vi "Find Specific USB Com Port.vi"(4 "Error In":errorcluster, 7 "Identifiers (regular expressions)":T2={"Vendor ID"="VID_0403", "Product ID"="PID_6001", "S/N"="FTXOVPUUA"}) -> (0 "Error Out":errorcluster, 2 "Device Info":T1={"Service"="FTSER2K", "Manufacturer"="FTDI", "PNPDeviceID"="FTDIBUS\\VID_0403+PID_6001+FTTR2S8CA\\0000"}, 3 "Com Port":refnum<visa-resource-name>)   [LabVIEW 2016]
uses:
  <vilib>/Utility/error.llb/Error Cluster From Error Code.vi
  <vilib>/ErrorRing/Error Ring.xnode
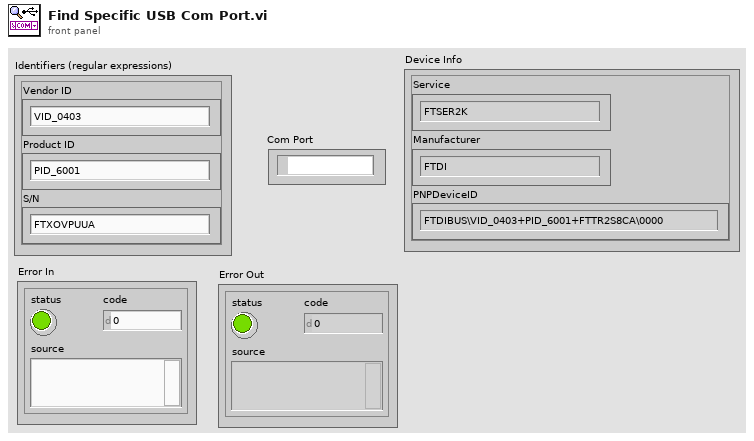
[diagram p1: front panel]
types:
  T1 = cluster{"Service":string, "Manufacturer":string, "PNPDeviceID":string}
  T2 = cluster{"Vendor ID":string, "Product ID":string, "S/N":string}
  T3 = cluster{"Service":string, "Manufacturer":string, "Device":string, "Vendor ID":string, "Product ID":string, "S/N":string, "Instance":string}
  T4 = cluster{"Service":string, "Manufacturer":string, "PNPDeviceID":string}[]
  T5 = cluster{"Name":string, "Caption":string, "Description":string}[]
  T6 = cluster{"Name":string, "Caption":string, "Description":string}
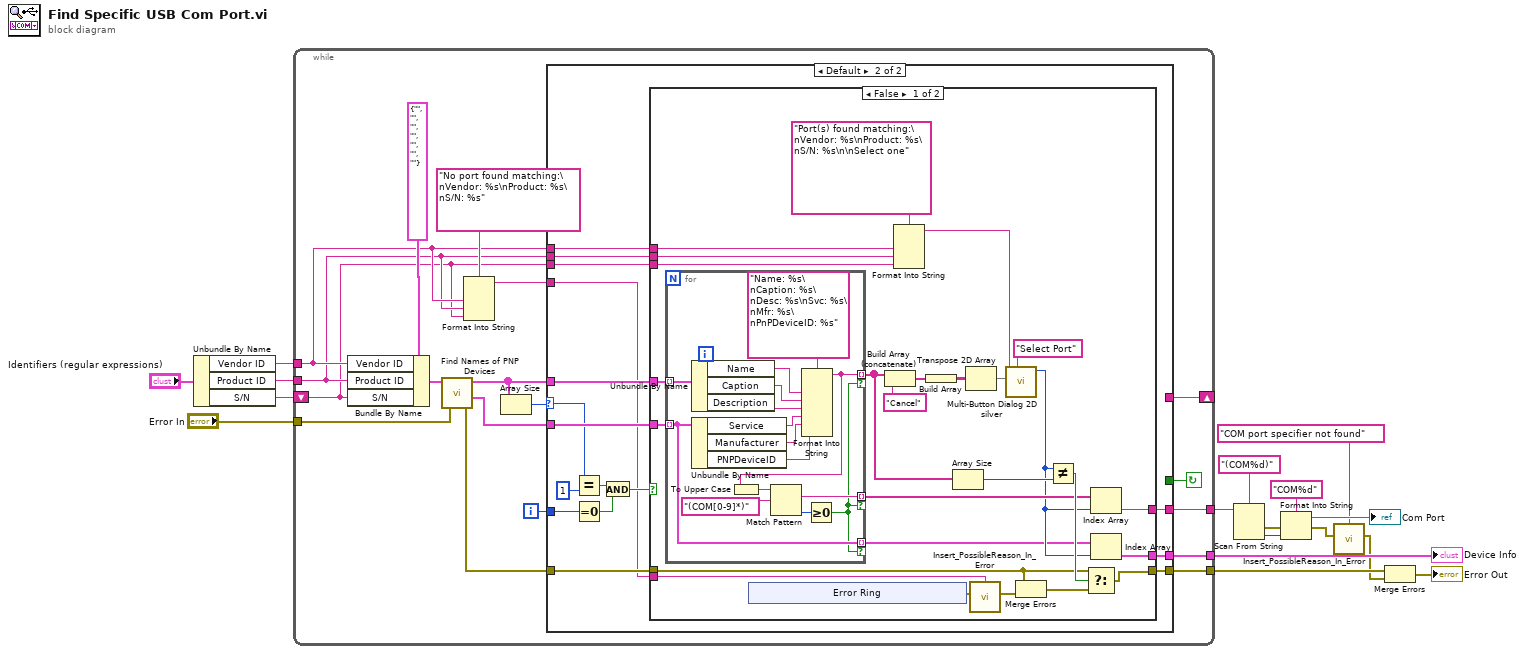
[diagram p0: block diagram]
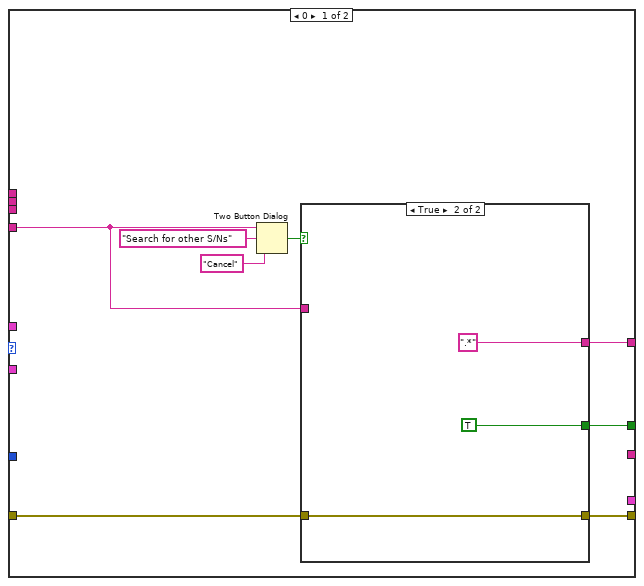
[diagram p2: hidden frame]
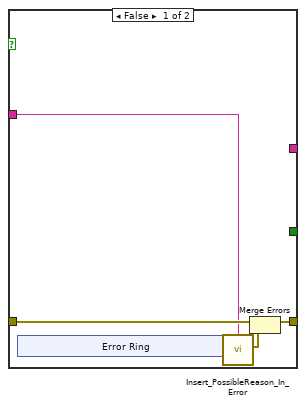
[diagram p3: hidden frame]
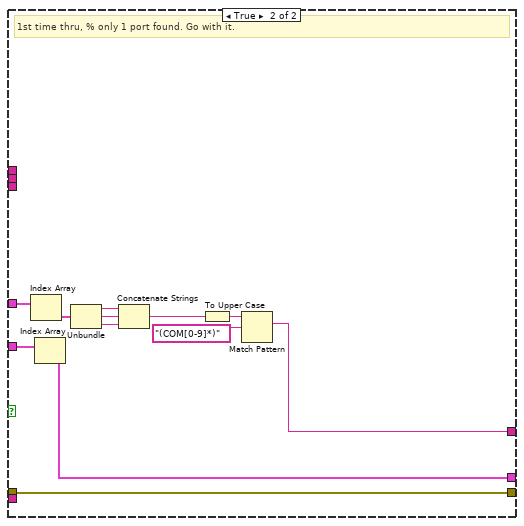
[diagram p4: hidden frame]
diagram:
  n1 = Unbundle By Name("Identifiers (regular expressions)") -> ("Vendor ID"=w15:string, "Product ID"=w14:string, "S/N"=w13:string)
  n2 = while {
    tunnel: "Error In" -> [w26]
    tunnel: w15 -> [w22]
    tunnel: w14 -> [w21]
    shift-right: [w31] -> _
    shift-left: w13 -> [w20]
    tunnel: [w29] -> w12
    tunnel: [w27] -> w11
    tunnel: [w18] -> w2
    i -> [w28]
    stop <- w30 continue-if-true
    n3 = Bundle By Name(cluster=T3 {"Service"="", "Manufacturer"="", "Device"="", "Vendor ID"="", "Product ID"="", "S/N"="", "Instance"=""} ("Identifiers (regular expressions)"), "Vendor ID"=w22, "Product ID"=w21, "S/N"=w20) -> (w34:T3)
    n4 = call "Find Names of PNP Devices.vi"("Error In"=w26, "Identifiers (regular expressions. Use blank to ignore)"=w34) -> ("Error Out"=w25:errorcluster, "Matching Items"=w24:T4, "Names"=w33:T5)  [unwired: 3 in]
    n5 = Format Into String(format string="No port found matching:\nVendor: %s\nProduct: %s\nS/N: %s", w22, w21, w20) -> (resulting string=w19:string)  [unwired: 2 in, 1 out]
    n6 = Array Size(array=w33) -> (size(s)=w32:i32)
    n7 = case shown="Default" w32 {
      selector: w32 -> [_ w65]
      tunnel: w33 -> [_ w68]
      tunnel: w22 -> [_ w71]
      tunnel: w21 -> [_ w70]
      tunnel: w20 -> [_ w69]
      tunnel: w24 -> [_ w67]
      tunnel: [w40 _] -> w31
      tunnel: [w39 _] -> w30
      tunnel: w25 -> [w38 w59]
      tunnel: [w37 w58] -> w29
      tunnel: w28 -> [_ w63]
      tunnel: [_ w60] -> w27
      tunnel: w19 -> [w36 w57]
      tunnel: [_ w56] -> w18
      frame 0 {
        n8 = Two Button Dialog(message=w36, 1:"Cancel" ("F button name (\"Cancel\")"), 2:"Search for other S/Ns" ("T button name (\"OK\")")) -> (T button?=w41:bool)
        n9 = case shown="True" w41 {
          tunnel: [_ ".*" ("S/N")] -> w40
          tunnel: [_ TRUE] -> w39
          tunnel: w38 -> [w48 w53]
          tunnel: [w44 w53] -> w37
          tunnel: w36 -> [w45 _]
          frame False {
            n10 = xnode "Error Ring"() -> ("error out"=w46:errorcluster)
            n11 = call "Insert_PossibleReason_In_Error.vi"("Possible Reason"=w45, "error in"=w46) -> ("error out"=w47:errorcluster)  [unwired: 6 in]
            n12 = Merge Errors(w48, w47) -> (w44:errorcluster)
          }
          frame True {
          }
        }
      }
      frame Default {
        n13 = Equal?(x=w65, y=1) -> (x = y?=w66:bool)
        n14 = Equal To 0?(x=w63) -> (x = 0?=w62:bool)
        n15 = And(x=w66, y=w62) -> (x .and. y?=w61:bool)
        n16 = case shown="False" w61 {
          tunnel: w71 -> [w95 _]
          tunnel: w70 -> [w94 _]
          tunnel: w69 -> [w93 _]
          tunnel: w68 -> [w90 w128]
          tunnel: w67 -> [w73 w127]
          tunnel: [w89 w126] -> w60
          tunnel: w59 -> [w79 w121]
          tunnel: [w77 w121] -> w58
          tunnel: w57 -> [w78 _]
          tunnel: [w74 w117] -> w56
          frame False {
            n17 = for {
              tunnel: w90 -> [w112] mode=indexing
              tunnel: w73 -> [w103] mode=indexing
              tunnel: [w106] -> w85 mode=indexing if=w102
              tunnel: [w104] -> w76 mode=indexing if=w102
              tunnel: [w103] -> w72 mode=indexing if=w102
              n18 = Unbundle By Name(w112) -> ("Name"=w111:string, "Caption"=w110:string, "Description"=w109:string)
              n19 = Unbundle By Name(w103) -> ("Service"=w115:string, "Manufacturer"=w114:string, "PNPDeviceID"=w113:string)
              n20 = Format Into String(format string="Name: %s\nCaption: %s\nDesc: %s\nSvc: %s\nMfr: %s\nPnPDeviceID: %s", w111, w110, w109, w115, w114, w113) -> (resulting string=w106:string)  [unwired: 2 in, 1 out]
              n21 = To Upper Case(1:w106) -> (0:w108:string)
              n22 = Match Pattern(string=w108, regular expression="(COM[0-9]*)") -> (match substring=w104:string, offset past match=w105:i32)  [unwired: 1 in, 2 out]
              n23 = Greater Or Equal To 0?(x=w105) -> (x >= 0?=w102:bool)
            }
            n24 = xnode "Error Ring"() -> ("error out"=w82:errorcluster)
            n25 = Build Array (concatenate)(w85, "Cancel" ("Title (blank)")) -> (w88:string[])
            n26 = Format Into String(format string="Port(s) found matching:\nVendor: %s\nProduct: %s\nS/N: %s\n\nSelect one", w95, w94, w93) -> (resulting string=w96:string)  [unwired: 2 in, 1 out]
            n27 = Build Array(w88) -> (w87:string[][])
            n28 = Array Size(array=w85) -> (size(s)=w84:i32)
            n29 = Transpose 2D Array(2D array=w87) -> (transposed array=w91:string[][])
            n30 = call "Insert_PossibleReason_In_Error.vi"("Possible Reason"=w78, "error in"=w82) -> ("error out"=w83:errorcluster)  [unwired: 6 in]
            n31 = call "Multi-Button Dialog 2D silver.vi"("Title (blank)"="Select Port", "Button Texts"=w91, "Message String"=w96) -> ("button row"=w75:i32)  [unwired: 4 in, 1 out]
            n32 = Merge Errors(w79, w83) -> (w80:errorcluster)
            n33 = Not Equal?(x=w75, y=w84) -> (x != y?=w81:bool)
            n34 = Select(t=w79, s=w81, f=w80) -> (s? t:f=w77:errorcluster)
            n35 = Index Array(array=w76, index=w75) -> (element=w74:string)
            n36 = Index Array(array=w72, index=w75) -> (element=w89:T1)
          }
          frame True {
            # "1st time thru, % only 1 port found. Go with it."
            n37 = Index Array(array=w128) -> (element=w125:T6)  [unwired: 1 in]
            n38 = Index Array(array=w127) -> (element=w126:T1)  [unwired: 1 in]
            n39 = Unbundle(w125) -> ("Name"=w124:string, "Caption"=w123:string, "Description"=w122:string)
            n40 = Concatenate Strings(w124, w123, w122) -> (w118:string)
            n41 = To Upper Case(1:w118) -> (0:w120:string)
            n42 = Match Pattern(string=w120, regular expression="(COM[0-9]*)") -> (match substring=w117:string)  [unwired: 1 in, 3 out]
          }
        }
      }
    }
  }
  "Device Info" <- w11
  n43 = Scan From String(format string="(COM%d)", input string=w2) -> (error out=w6:errorcluster, output 1=w9:i32)  [unwired: 3 in, 2 out]
  n44 = Format Into String(format string="COM%d", error in=w6, w9) -> (resulting string=→"Com Port":string, error out=w5:errorcluster)  [unwired: 1 in]
  n45 = call "Insert_PossibleReason_In_Error.vi"("Possible Reason"="COM port specifier not found", "error in"=w5) -> ("error out"=w3:errorcluster)  [unwired: 6 in]
  n46 = Merge Errors(w12, w3) -> (→"Error Out":errorcluster)
